vi "Numerical Conversion.vi"(7 "width":i32=4, 11 "num":i32) -> (3 "字符串":string)   [LabVIEW 2014]
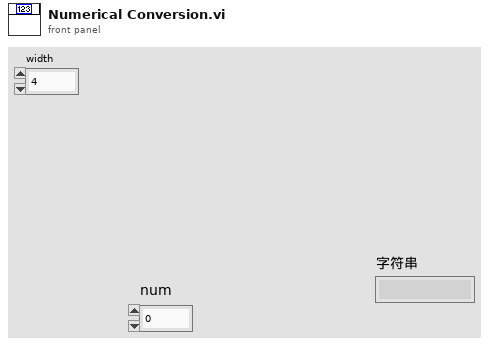
[diagram p1: front panel]
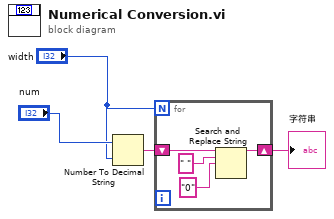
[diagram p0: block diagram]
diagram:
  n1 = Number To Decimal String(number="num", width (-)="width") -> (decimal integer string=w4:string)
  n2 = for {
    N: "width" -> [_]
    shift-right: [w5] -> w3
    shift-left: w4 -> [w8]
    n3 = Search and Replace String(input string=w8, search string=" " ("搜索字符串"), replace string="0" ("替换字符串(\"\")")) -> (result string=w5:string)  [unwired: 1 in, 7 out]
  }
  "字符串" <- w3
